vi "write header.vi"(7 "number of samples for this channel":u32, 8 "error in (no error)":errorcluster, 9 "pos offset (bytes:0)":i32, 10 "Channel name":string, 11 "Ref Num":refnum<file>) -> (0 "error out":errorcluster, 1 "mark after write (bytes)":i32, 3 "Dup Ref Num":refnum<file>)   [LabVIEW 2015]
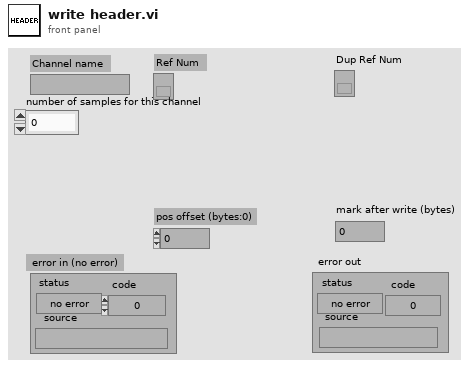
[diagram p1: front panel]
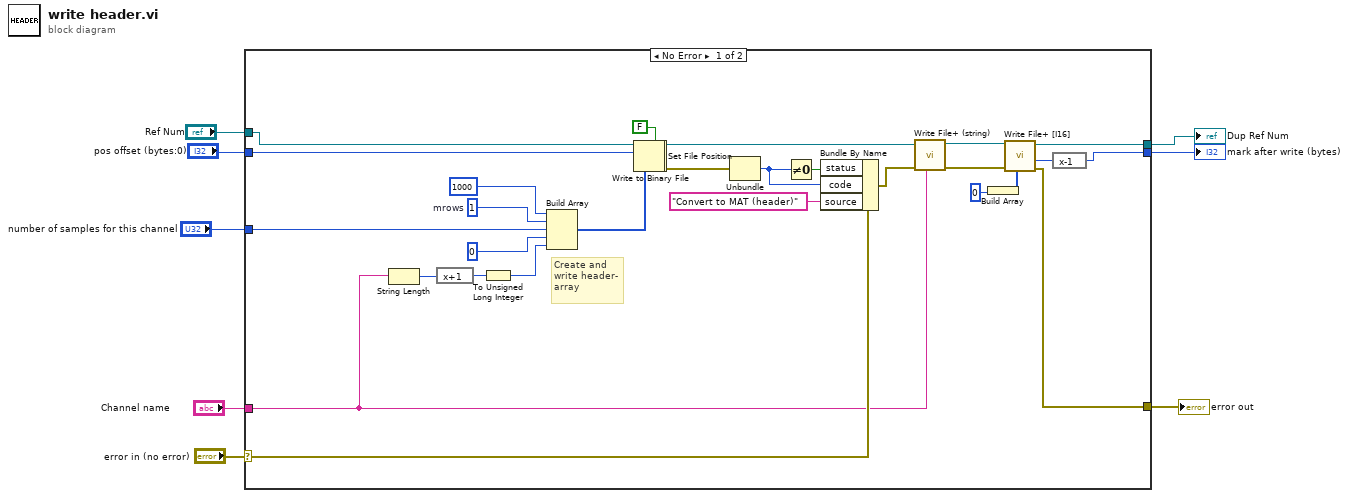
[diagram p0: block diagram]
diagram:
  n1 = case shown="No Error" "error in (no error)" {
    selector: "error in (no error)" -> [w20 w38]
    tunnel: [w9 w38] -> w8
    tunnel: [w11 w40] -> w6
    tunnel: "Ref Num" -> [w29 w40]
    tunnel: [w10 -1] -> w5
    tunnel: "Channel name" -> [w17 _]
    tunnel: "pos offset (bytes:0)" -> [w14 _]
    tunnel: "number of samples for this channel" -> [w12 _]
    frame No Error {
      w25 = u32 1  # mrows
      # "Create and\nwrite header-\narray"
      n2 = String Length(string=w17) -> (length=w16:i32)
      n3 = expression code="x+1"(w16) -> (w15:i32)
      n4 = To Unsigned Long Integer(number=w15) -> (unsigned 32bit integer=w35:u32)
      n5 = Build Array(u32 1000, w25, w12, u32 0, w35) -> (w28:u32[])
      n6 = Set File Position(offset (in bytes) (0)=w14, refnum=w29) -> (refnum out=w23:refnum<file>, error out=w22:errorcluster)  [unwired: 2 in]
      n7 = Write to Binary File(file (use dialog)=w23, data=w28, error in=w22, 5:FALSE ("prepend array or string size? (T)")) -> (refnum out=w34:refnum<file>, error out=w27:errorcluster)  [unwired: 2 in, 1 out]
      n8 = Unbundle(w27) -> ("code"=w24:i32)  [unwired: 2 out]
      n9 = Not Equal To 0?(x=w24) -> (x != 0?=w37:bool)
      n10 = Bundle By Name(cluster=w20, "status"=w37, "code"=w24, "source"="Convert to MAT (header)") -> (w26:errorcluster)
      n11 = call <vilib>:"Write File+ (string).vi"("string"=w17, "error in (no error)"=w26, "refnum"=w34) -> ("error out"=w31:errorcluster, "dup refnum"=w30:refnum<file>)  [unwired: 4 in, 1 out]
      n12 = Build Array(u8 0) -> (w33:u8[])
      n13 = call <vilib>:"Write File+ [I16].vi"("1D array"=w33, "error in (no error)"=w31, "refnum"=w30) -> ("error out"=w9:errorcluster, "mark after write (bytes)"=w13:i32, "dup refnum"=w11:refnum<file>)  [unwired: 6 in]
      n14 = expression code="x-1"(w13) -> (w10:i32)
    }
    frame Error {
    }
  }
  "Dup Ref Num" <- w6
  "error out" <- w8
  "mark after write (bytes)" <- w5
